vi "Perform Action.vi"(8 "error in (no error)":errorcluster, 10 "Input":variant, 11 "FGen PXI Std Waveform CFG in":refnum<class "FGen PXI Std Waveform CFG.lvclass">) -> (0 "error out":errorcluster, 2 "Output":variant, 3 "FGen PXI Std Waveform CFG out":refnum<class "FGen PXI Std Waveform CFG.lvclass">)   [LabVIEW 2023, in "FGen PXI Std Waveform CFG.lvlib" / "FGen PXI Std Waveform CFG.lvclass"]
uses:
  FGen PXI Std Waveform CFG.lvclass
  Std Waveform Action Pams.ctl
  FGen PXI Base CFG/FGen PXI Base CFG.lvclass/FGen PXI Base CFG.ctl
  FGen PXI Base CFG/FGen PXI Base CFG.lvclass
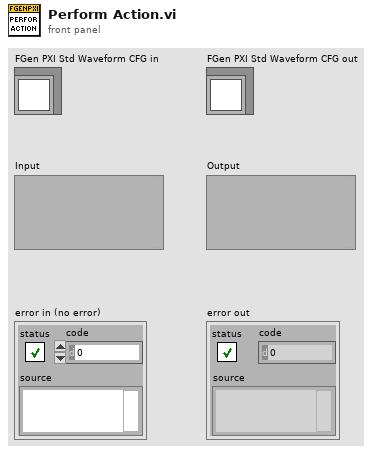
[diagram p1: front panel]
types:
  T1 = typedef "FGen PXI Std Waveform CFG.lvlib/FGen PXI Std Waveform CFG.lvclass/Std Waveform Action Pams.ctl" = cluster{"Frequency":dbl, "Amplitude":dbl, "DC Offset":dbl}
  T2 = cluster{"Channel":string, "Std Waveform Action Pams":T1}
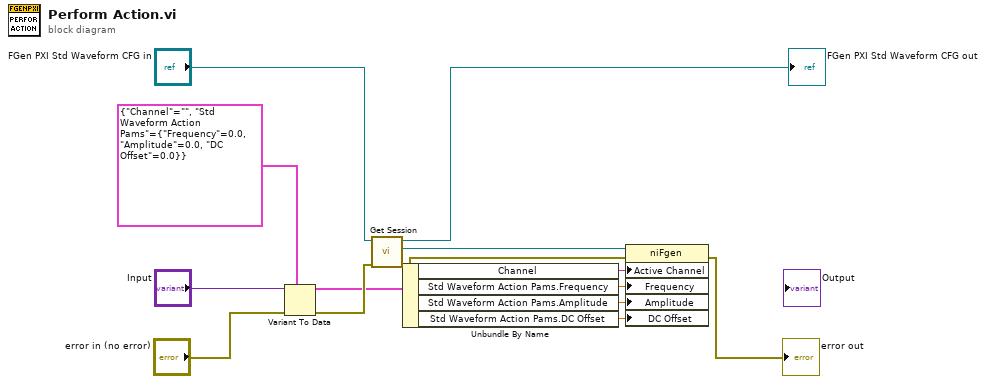
[diagram p0: block diagram]
diagram:
  n1 = Variant To Data(error in="error in (no error)", type=T2 {"Channel"="", "Std Waveform Action Pams"={"Frequency"=0.0, "Amplitude"=0.0, "DC Offset"=0.0}}, Variant="Input") -> (data=w8:T2, error out=w11:errorcluster)
  n2 = call "Get Session.vi"("error in (no error)"=w11, "FGen PXI Base CFG in"="FGen PXI Std Waveform CFG in") -> ("error out"=w3:errorcluster, "Session"=w14:refnum<k15>, "FGen PXI Base CFG out"=→"FGen PXI Std Waveform CFG out":refnum<class "FGen PXI Std Waveform CFG.lvclass">)  [unwired: 7 in]
  n3 = Unbundle By Name(w8) -> ("Channel"=w7:string, "Std Waveform Action Pams.Frequency"=w6:dbl, "Std Waveform Action Pams.Amplitude"=w5:dbl, "Std Waveform Action Pams.DC Offset"=w4:dbl)
  n4 = property class="niFgen"(reference=w14, error in=w3, "Active Channel"=w7, "Frequency"=w6, "Amplitude"=w5, "DC Offset"=w4) -> (error out=→"error out":errorcluster)  [unwired: 1 out]
